vi "SetServiceArrayInputs.vi"(8 "error in":errorcluster, 10 "Properties":string[][](array[string]), 11 "Thing Info In":T2) -> (0 "error out":errorcluster, 3 "Thing Info Out":T2)   [LabVIEW 2015]
uses:
  <vilib>/httpClient/ClientHandle.ctl
  <vilib>/httpClient/POSTBuffer.vi
  <vilib>/httpClient/LabVIEWHTTPClient.lvlib
panel:
  out "final url":string
  out "reply body":string
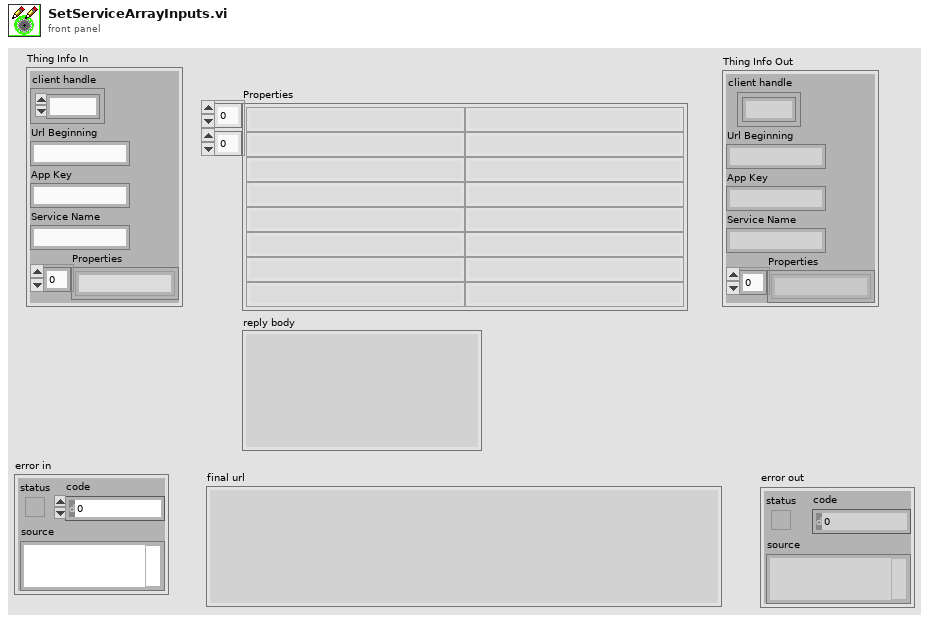
[diagram p1: front panel]
types:
  T1 = typedef "LabVIEWHTTPClient.lvlib/ClientHandle.ctl" = refnum<k1>
  T2 = cluster{"client handle":T1, "Url Beginning":string, "App Key":string, "Service Name":string, "Properties":string[]}
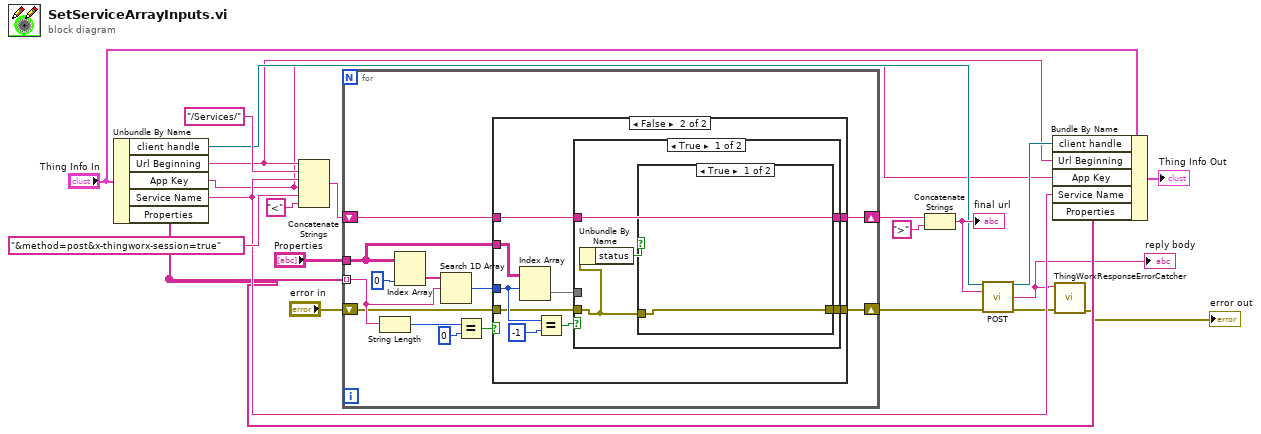
[diagram p0: block diagram]
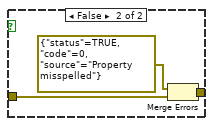
[diagram p3: hidden frame]
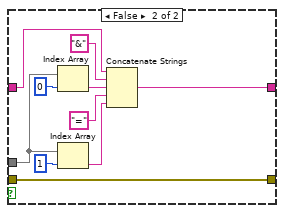
[diagram p4: hidden frame]
diagram:
  n1 = Unbundle By Name("Thing Info In") -> ("client handle"=w11:T1, "Url Beginning"=w9:string, "App Key"=w4:string, "Service Name"=w6:string, "Properties"=w5:string[])
  n2 = Concatenate Strings(w9, "/Services/" ("string"), w6, w4, "&method=post&x-thingworx-session=true" ("string"), "<" ("string")) -> (w18:string)
  n3 = for {
    tunnel: "Properties" -> [w31]
    shift-right: [w32] -> w17
    shift-left: w18 -> [w33]
    tunnel: w5 -> [w27] mode=indexing
    shift-right: [w22] -> w12
    shift-left: "error in" -> [w23]
    n4 = String Length(string=w27) -> (length=w26:i32)
    n5 = Index Array(array=w31, index (col)=0 ("disabled index (col)")) -> (element=w29:string[])  [unwired: 1 in]
    n6 = Search 1D Array(1D array=w29, element=w27) -> (index of element=w28:i32)  [unwired: 1 in]
    n7 = Equal?(x=w26, y=0) -> (x = y?=w24:bool)
    n8 = case shown="False" w24 {
      tunnel: w33 -> [w35 w44]
      tunnel: [w35 w43] -> w32
      tunnel: w31 -> [_ w41]
      tunnel: w28 -> [_ w40]
      tunnel: w23 -> [w34 w37]
      tunnel: [w34 w36] -> w22
      frame True {
      }
      frame False {
        n9 = Index Array(array=w41, index (row)=w40) -> (element=w39:string[])  [unwired: 1 in]
        n10 = Equal?(x=w40, y=-1) -> (x = y?=w38:bool)
        n11 = case shown="True" w38 {
          tunnel: w44 -> [w47 w61]
          tunnel: [w47 w59] -> w43
          tunnel: w39 -> [_ w58]
          tunnel: w37 -> [w46 w53]
          tunnel: [w48 w53] -> w36
          frame True {
            n12 = Unbundle By Name(w46) -> ("status"=w45:bool)
            n13 = case shown="True" w45 {
              tunnel: w46 -> [w49 w52]
              tunnel: [w49 w50] -> w48
              frame True {
              }
              frame False {
                n14 = Merge Errors(errorcluster {"status"=TRUE, "code"=0, "source"="Property misspelled"} ("error in"), w52) -> (w50:errorcluster)
              }
            }
          }
          frame False {
            n15 = Index Array(array=w58, index=0) -> (element=w55:string)
            n16 = Index Array(array=w58, index=1) -> (element=w57:string)
            n17 = Concatenate Strings(w61, "&" ("string"), w55, "=" ("string"), w57) -> (w59:string)
          }
        }
      }
    }
  }
  n18 = Concatenate Strings(w17, ">" ("string")) -> (w16:string)
  "final url" <- w16
  n19 = call-poly <vilib>:"POST.vi"("client handle"=w11, "url"=w16, "error in (no error)"=w12) -> ("client handle out"=w10:T1, "body"=w2:string, "error out"=w3:errorcluster)  [unwired: 9 in, 1 out]
  "reply body" <- w2
  n20 = Bundle By Name(cluster="Thing Info In", "client handle"=w10, "Url Beginning"=w9, "App Key"=w4, "Service Name"=w6, "Properties"=w5) -> (→"Thing Info Out":T2)
  n21 = call "ThingWorxResponseErrorCatcher.vi"("error in (no error)"=w3, "body"=w2) -> ("error out"=→"error out":errorcluster)  [unwired: 9 in]
